vi "Write to VULTR using STD VIs.vi"(0 "DayCode":string, 1 "conninfo":path, 5 "Voltage":dbl format="%#_13g", 7 "Table":string="APA.Frequency_Table", 9 "SQL query":string="SELECT PhaseNoiseID\nFROM APA.PhaseNoise_Table \nORDER BY \nPhaseNoiseID DESC \nLIMIT 1", 11 "error in (no error)":errorcluster, 12 "UnitID":i32) -> (4 "Get ID":i32, 15 "error out":errorcluster)   [LabVIEW 2017]
uses:
  <vilib>/addons/database/Connection.llb/Conn ObjectReference.ctl
  <vilib>/addons/database/Auxilliary.llb/DB Tools Format Datetime String (Time Stamp).vi
  <vilib>/addons/database/Connection.llb/DB Tools Open Connec (Path).vi
  <vilib>/addons/database/Connection.llb/Conn Execute.vi
  <vilib>/addons/database/Recordset.llb/Rec Fetch Recordset Data (R).vi
  <vilib>/addons/database/Recordset.llb/Rec Destroy - Connection.vi
  <vilib>/addons/database/NI_Database_API.lvlib
panel:
  in  "FrequencyID":i32
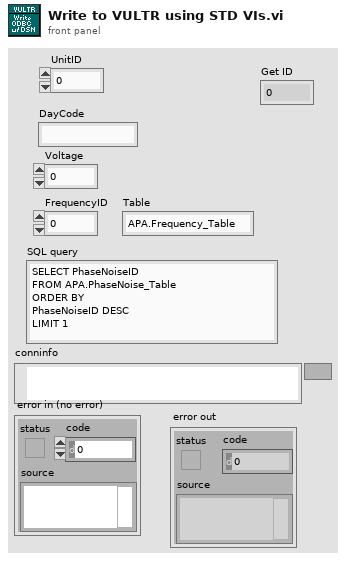
[diagram p1: front panel]
types:
  T1 = typedef "NI_Database_API.lvlib/Conn ObjectReference.ctl" = refnum<k1>
  T2 = enum16{"Test Ping", "Open Dbase", "Write Dbase", "Close Dbase", "Open Local", "Write Local", "Close Local", "Exit"}
  T3 = cluster{"date/time string":string, "UnitID":i32, "DayCode":string, "Voltage":dbl}
  T4 = cluster{"conninfo":path, "conn":T1, "refnum":refnum<file>}
  T5 = typedef "NI_Database_API.lvlib/Rec ObjectReference.ctl" = refnum<k1>
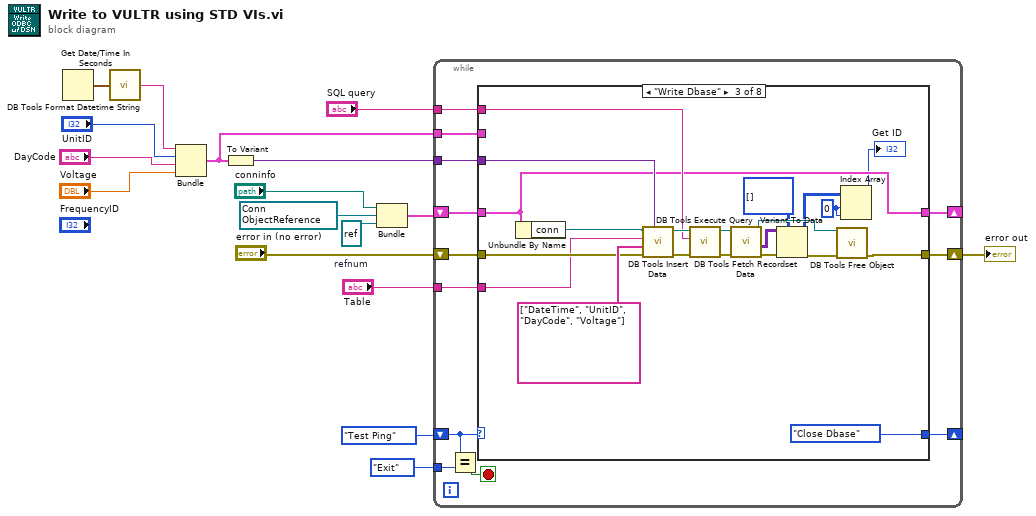
[diagram p0: block diagram]
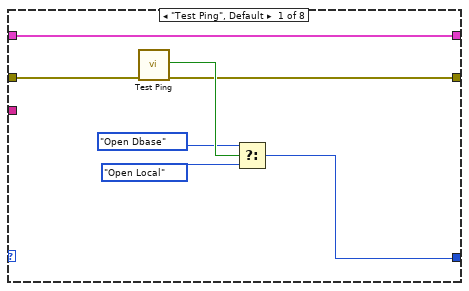
[diagram p2: hidden frame]
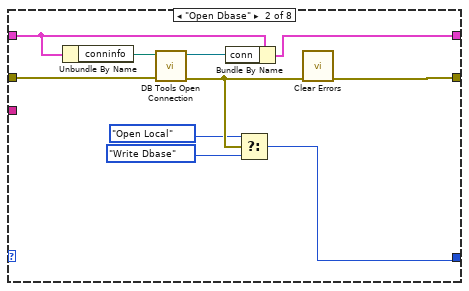
[diagram p3: hidden frame]
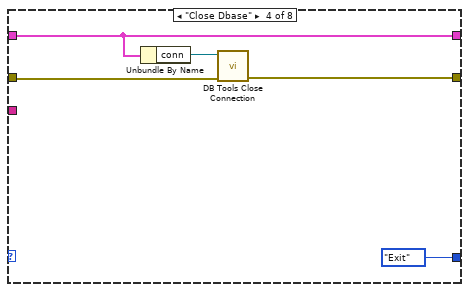
[diagram p4: hidden frame]
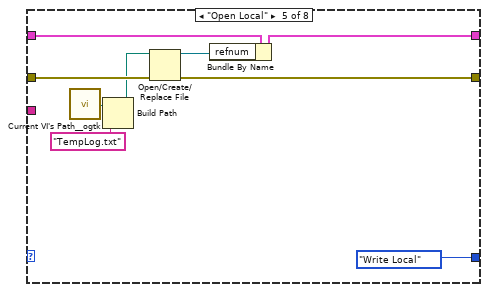
[diagram p5: hidden frame]
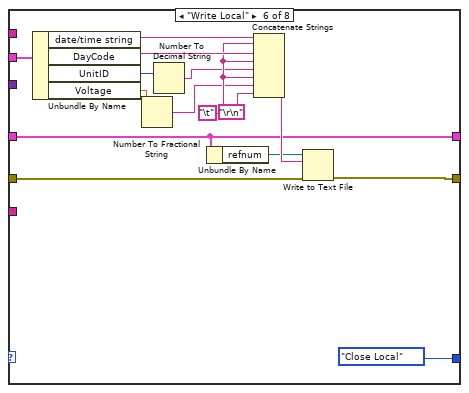
[diagram p6: hidden frame]
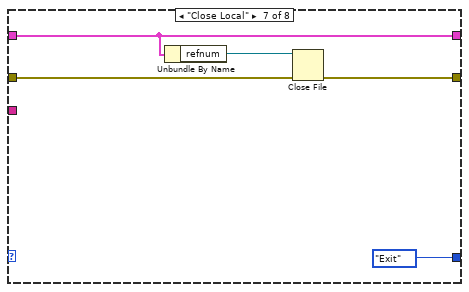
[diagram p7: hidden frame]
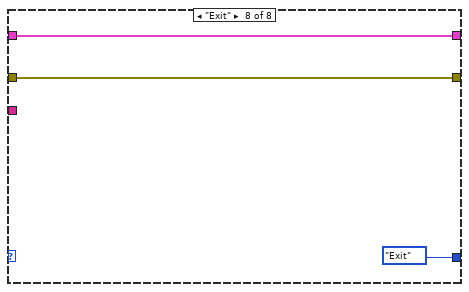
[diagram p8: hidden frame]
diagram:
  w4 = refnum<file> refnum  # refnum
  w10 = T1 refnum items=["Connection"] ("conn")
  n1 = Get Date/Time In Seconds() -> (seconds since 1Jan1904=w16:timestamp)
  n2 = call-poly <vilib>:"DB Tools Format Datetime String.vi"("time stamp"=w16) -> ("date/time string"=w15:string)
  n3 = Bundle("date/time string"=w15, "UnitID"="UnitID", "DayCode"="DayCode", "Voltage"="Voltage") -> (w5:T3)  [unwired: 1 in]
  n4 = To Variant(anything=w5) -> (Variant=w8:variant)
  n5 = Bundle("conninfo"="conninfo", "conn"=w10, "refnum"=w4) -> (w9:T4)  [unwired: 1 in]
  n6 = while {
    shift-right: [w25] -> _
    shift-left: T2."Test Ping" ("Enum") -> [w29]
    tunnel: T2."Exit" ("Enum") -> [w28]
    shift-right: [w20] -> w6
    shift-left: "error in (no error)" -> [w26]
    shift-right: [w23] -> _
    shift-left: w9 -> [w24]
    tunnel: w8 -> [w22]
    tunnel: "SQL query" -> [w21]
    tunnel: w5 -> [w19]
    tunnel: "Table" -> [w18]
    stop <- w27 stop-if-true
    n7 = Equal?(x=w29, y=w28) -> (x = y?=w27:bool)
    n8 = case shown="\"Write Dbase\"" w29 {
      tunnel: w26 -> [w36 w46 w55 w72 w79 w90 w100 w102]
      tunnel: [w32 w45 T2."Close Dbase" ("Enum") T2."Exit" ("Enum") T2."Write Local" ("Enum") T2."Close Local" ("Enum") T2."Exit" ("Enum") T2."Exit" ("Enum")] -> w25
      tunnel: w24 -> [w31 w42 w51 w71 w81 w87 w98 w104]
      tunnel: [w31 w40 w51 w71 w74 w87 w98 w104] -> w23
      tunnel: w22 -> [_ _ w53 _ _ _ _ _]
      tunnel: w21 -> [_ _ w52 _ _ _ _ _]
      tunnel: [w30 w39 w49 w68 w75 w89 w99 w102] -> w20
      tunnel: w19 -> [_ _ _ _ _ w91 _ _]
      tunnel: w18 -> [_ _ w47 _ _ _ _ _]
      frame "Test Ping", Default {
        n9 = call "Test Ping.vi"("error in (no error)"=w36) -> ("error out"=w30:errorcluster, "x = y?"=w35:bool)  [unwired: 9 in]
        n10 = Select(t=T2."Open Dbase" ("Enum"), s=w35, f=T2."Open Local" ("Enum")) -> (s? t:f=w32:T2)
      }
      frame "Open Dbase" {
        n11 = Unbundle By Name(w42) -> ("conninfo"=w43:path)
        n12 = call-poly <vilib>:"DB Tools Open Connection.vi"("error in (no error)"=w46, "connection information"=w43) -> ("error out"=w44:errorcluster, "connection reference"=w41:T1)  [unwired: 6 in]
        n13 = Bundle By Name(cluster=w42, "conn"=w41) -> (w40:T4)
        n14 = Select(t=T2."Open Local" ("Enum"), s=w44, f=T2."Write Dbase" ("Enum")) -> (s? t:f=w45:T2)
        n15 = call <vilib>:"Clear Errors.vi"("error in (no error)"=w44) -> ("error out"=w39:errorcluster)  [unwired: 5 in, 1 out]
      }
      frame "Write Dbase" {
        w59 = 0 ("index (row)")
        n16 = Unbundle By Name(w51) -> ("conn"=w54:T1)
        n17 = call <vilib>:"DB Tools Insert Data.vi"("data"=w53, "error in (no error)"=w55, "columns"=string[] ["DateTime", "UnitID", "DayCode", "Voltage"], "table"=w47, "connection reference"=w54) -> ("error out"=w61:errorcluster, "connection reference out"=w60:T1)  [unwired: 5 in]
        n18 = call-poly <vilib>:"DB Tools Execute Query.vi"("error in (no error)"=w61, "SQL query"=w52, "connection reference"=w60) -> ("error out"=w63:errorcluster, "recordset reference"=w62:T5)  [unwired: 5 in]
        n19 = call-poly <vilib>:"DB Tools Fetch Recordset Data.vi"("error in (no error)"=w63, "recordset reference"=w62) -> ("error out"=w65:errorcluster, "recordset data"=w64:variant[][], "recordset reference out"=w66:T5)  [unwired: 3 in]
        n20 = Variant To Data(error in=w65, type=i32[][] [], Variant=w64) -> (data=w58:i32[][], error out=w67:errorcluster)
        n21 = call-poly <vilib>:"DB Tools Free Object.vi"("error in (no error)"=w67, "recordset reference"=w66) -> ("error out"=w49:errorcluster)  [unwired: 8 in, 1 out]
        n22 = Index Array(array=w58, index (row)=w59, index (col)=w59) -> (element=→"Get ID":i32)
      }
      frame "Close Dbase" {
        n23 = Unbundle By Name(w71) -> ("conn"=w70:T1)
        n24 = call <vilib>:"DB Tools Close Connection.vi"("error in (no error)"=w72, "connection reference"=w70) -> ("error out"=w68:errorcluster)  [unwired: 5 in]
      }
      frame "Open Local" {
        n25 = call <userlib>:"Current VI's Path__ogtk.vi"() -> ("Current VI's Path (+ Relative)"=w78:path)  [unwired: 1 in]
        n26 = Build Path(base path=w78, name or relative path="TempLog.txt") -> (appended path=w76:path)
        n27 = Open/Create/Replace File(file path (use dialog)=w76, error in=w79) -> (refnum out=w73:refnum<file>, error out=w75:errorcluster)  [unwired: 4 in, 1 out]
        n28 = Bundle By Name(cluster=w81, "refnum"=w73) -> (w74:T4)
      }
      frame "Write Local" {
        w93 = "\t"
        n29 = Unbundle By Name(w91) -> ("date/time string"=w95:string, "DayCode"=w94:string, "UnitID"=w85:i32, "Voltage"=w83:dbl)
        n30 = Number To Fractional String(number=w83) -> (F-format string=w82:string)  [unwired: 3 in]
        n31 = Number To Decimal String(number=w85) -> (decimal integer string=w84:string)  [unwired: 1 in]
        n32 = Unbundle By Name(w87) -> ("refnum"=w86:refnum<file>)
        n33 = Concatenate Strings(w95, w93, w94, w93, w84, w93, w82, "\r\n") -> (w88:string)
        n34 = Write to Text File(file (use dialog)=w86, text=w88, error in=w90) -> (error out=w89:errorcluster)  [unwired: 1 in, 2 out]
      }
      frame "Close Local" {
        n35 = Unbundle By Name(w98) -> ("refnum"=w97:refnum<file>)
        n36 = Close File(refnum=w97, error in=w100) -> (error out=w99:errorcluster)  [unwired: 1 out]
      }
      frame "Exit" {
      }
    }
  }
  "error out" <- w6
